vi "Find Node.vi"(7 "Create?":bool, 8 "error in (no error)":errorcluster, 10 "Tokens":string[](array[string]), 11 "PathTree in":refnum<class "PathTree.lvclass">) -> (0 "error out":errorcluster, 2 "Node":refnum<class "PathTreeNode.lvclass">, 3 "PathTree out":refnum<class "PathTree.lvclass">)   [LabVIEW 2020, in "Advanced Structures.lvlib" / "PathTree.lvclass"]
uses:
  PathTree.lvclass
  PathTreeNode/PathTreeNode.lvclass
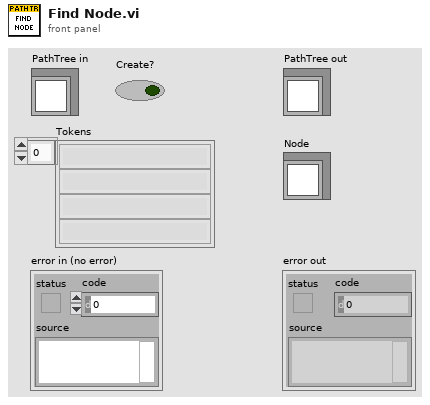
[diagram p1: front panel]
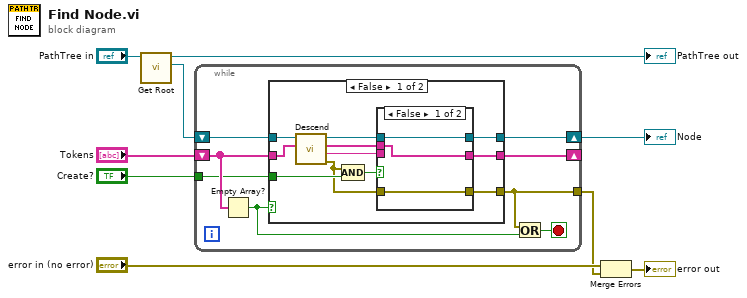
[diagram p0: block diagram]
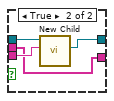
[diagram p2: hidden frame]
diagram:
  n1 = call "Get Root.vi"("PathTree in"="PathTree in") -> ("Root"=w7:refnum<class "PathTreeNode.lvclass">, "PathTree out"=→"PathTree out":refnum<class "PathTree.lvclass">)  [unwired: 8 in, 1 out]
  n2 = while {
    shift-right: [w13] -> _
    shift-left: "Tokens" -> [w17]
    shift-right: [w14] -> w3
    shift-left: w7 -> [w15]
    tunnel: [w11] -> w4
    tunnel: "Create?" -> [w10]
    stop <- w12 stop-if-true
    n3 = Empty Array?(array=w17) -> (empty?=w16:bool)
    n4 = case shown="False" w16 {
      tunnel: w17 -> [w27 w36]
      tunnel: w15 -> [w28 w37]
      tunnel: [w20 w37] -> w14
      tunnel: [w21 w36] -> w13
      tunnel: [w18 _] -> w11
      tunnel: w10 -> [w26 _]
      frame False {
        n5 = call "Descend.vi"("Path Tokens"=w27, "PathTreeNode in"=w28) -> ("error out"=w19:errorcluster, "Child Token"=w24:string, "Remaining Tokens"=w23:string[], "PathTreeNode out"=w22:refnum<class "PathTreeNode.lvclass">)  [unwired: 6 in]
        n6 = Compound Arithmetic op=AND(w19, w26) -> (w25:bool)
        n7 = case shown="False" w25 {
          tunnel: w24 -> [_ w34]
          tunnel: w23 -> [w31 w33]
          tunnel: w22 -> [w30 w35]
          tunnel: [w31 w33] -> w21
          tunnel: [w30 w32] -> w20
          tunnel: w19 -> [w29 _]
          tunnel: [w29 _] -> w18
          frame False {
          }
          frame True {
            n8 = call "New Child.vi"("Child Token"=w34, "PathTreeNode in"=w35) -> ("Child"=w32:refnum<class "PathTreeNode.lvclass">)  [unwired: 7 in, 2 out]
          }
        }
      }
      frame True {
      }
    }
    n9 = Or(x=w11, y=w16) -> (x .or. y?=w12:bool)
  }
  "Node" <- w3
  n10 = Merge Errors("error in (no error)", w4) -> (→"error out":errorcluster)
